vi "CH_LM Measurement Abort.vi"(0 "Meter Index":i32, 5 "error in (no error)":errorcluster, 7 "Timeout / ms (3000)":i32=3000, 9 "Lock Timeout / ms (1000)":i32=1000) -> (11 "Lock timed out":bool, 14 "Meter Index":i32, 19 "error out":errorcluster)   [LabVIEW 2017, in "CH_LM.lvlib"]
doc: "This VI disables the streaming mode and flushes the read buffer.\n\n<B>Hint:</B> The USB Binary Data Streaming will be disabled with this command."
uses:
  CH_LM.lvlib
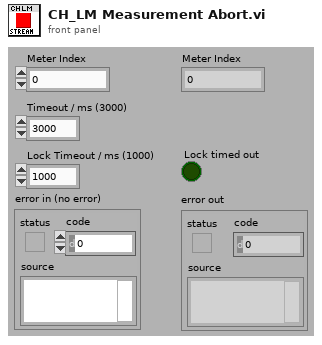
[diagram p1: front panel]
types:
  T1 = typedef "CH_LM.lvlib/CH_LM Communication Mode.ctl" = enum16{"None", "USB", "GPIB", "RS232"}
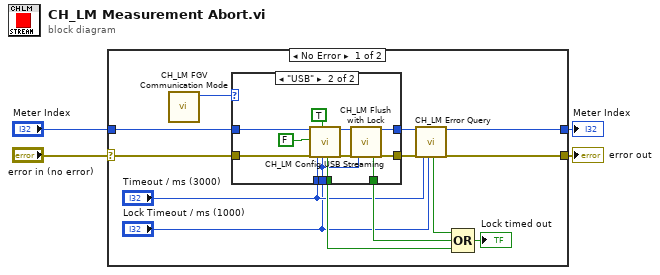
[diagram p0: block diagram]
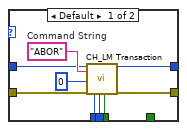
[diagram p2: hidden frame]
diagram:
  n1 = case shown="No Error" "error in (no error)" {
    selector: "error in (no error)" -> [w5 w40]
    tunnel: [w9 w40] -> w4
    tunnel: "Meter Index" -> [w6 w39]
    tunnel: [w8 w39] -> w1
    frame No Error {
      n2 = call "CH_LM FGV Communication Mode.vi"() -> ("Communication Mode"=w7:T1)  [unwired: 3 in, 5 out]
      n3 = case shown="\"USB\"" w7 {
        tunnel: [w19 w34] -> w16
        tunnel: [w18 w33] -> w15
        tunnel: [w20 w32] -> w14
        tunnel: [_ w31] -> w12
        tunnel: "Timeout / ms (3000)" -> [w22 w30]
        tunnel: "Lock Timeout / ms (1000)" -> [w21 w29]
        tunnel: w6 -> [w24 w28]
        tunnel: w5 -> [w23 w27]
        frame Default {
          w25 = "ABOR"  # Command String
          n4 = call "CH_LM Transaction.vi"("Meter Index"=w24, "Command String"=w25, "NofStrings (-1:all)"=0, "error in (no error)"=w23, "Timeout / ms (3000)"=w22, "Lock Timeout / ms (1000)"=w21) -> ("Lock timed out"=w20:bool, "Meter Index"=w19:i32, "error out"=w18:errorcluster)  [unwired: 11 out]
        }
        frame "USB" {
          n5 = call "CH_LM Config USB Streaming.vi"("Meter Index"=w28, "USB Streaming (disable)"=FALSE, "error in (no error)"=w27, "Timeout / ms (3000)"=w30, "Action (query)"=TRUE, "Lock Timeout / ms (1000)"=w29) -> ("Lock timed out"=w32:bool, "Meter Index"=w36:i32, "error out"=w35:errorcluster)  [unwired: 11 out]
          n6 = call "CH_LM Flush with Lock.vi"("Meter Index"=w36, "error in (no error)"=w35, "Lock Timeout / ms (1000)"=w29) -> ("Lock timed out"=w31:bool, "Meter Index"=w34:i32, "error out"=w33:errorcluster)  [unwired: 14 out]
        }
      }
      n7 = call "CH_LM Error Query.vi"("Meter Index"=w16, "error in (no error)"=w15, "Timeout / ms (3000)"="Timeout / ms (3000)", "Lock Timeout / ms (1000)"="Lock Timeout / ms (1000)") -> ("Lock timed out"=w13:bool, "Meter Index"=w8:i32, "error out"=w9:errorcluster)  [unwired: 13 out]
      n8 = Compound Arithmetic op=OR(w13, w12, w14) -> (→"Lock timed out":bool)
    }
    frame Error {
    }
  }
  "error out" <- w4
  "Meter Index" <- w1
